vi "Loss_calc.vi"(6 "Weight Regularizers":enum32{"None", "L1", "L2"}(radio), 7 "Weights":dbl[](array[numeric]), 9 "Loss Type":enum16{"MSE", "MAE"}(ring)=enum."MAE", 10 "Target":dbl, 11 "Data":dbl) -> (3 "Loss":dbl)   [LabVIEW 2019]
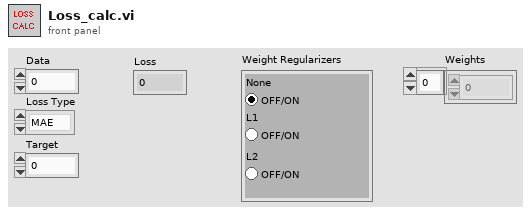
[diagram p1: front panel]
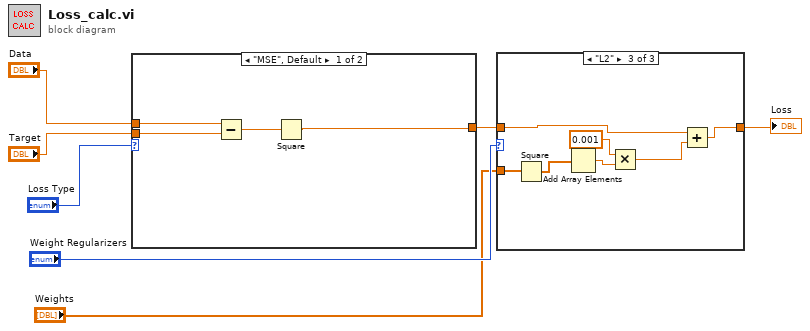
[diagram p0: block diagram]
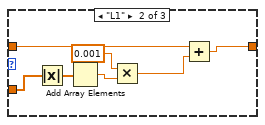
[diagram p3: hidden frame]
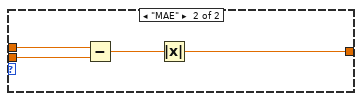
[diagram p4: hidden frame]
diagram:
  n1 = case shown="\"MSE\", Default" "Loss Type" {
    tunnel: "Data" -> [w11 w15]
    tunnel: "Target" -> [w10 w14]
    tunnel: [w8 w12] -> w3
    frame "MSE", Default {
      n2 = Subtract(x=w11, y=w10) -> (x-y=w9:dbl)
      n3 = Square(x=w9) -> (x^2=w8:dbl)
    }
    frame "MAE" {
      n4 = Subtract(x=w15, y=w14) -> (x-y=w13:dbl)
      n5 = Absolute Value(x=w13) -> (abs(x)=w12:dbl)
    }
  }
  n6 = case shown="\"L2\"" "Weight Regularizers" {
    tunnel: w3 -> [w16 w23 w27]
    tunnel: [w16 w17 w26] -> w2
    tunnel: "Weights" -> [_ w22 w25]
    frame "None", Default {
    }
    frame "L1" {
      n7 = Absolute Value(x=w22) -> (abs(x)=w18:dbl[])
      n8 = Add Array Elements(numeric array=w18) -> (sum=w19:dbl)
      n9 = Multiply(x=0.001, y=w19) -> (x*y=w20:dbl)
      n10 = Add(x=w23, y=w20) -> (x+y=w17:dbl)
    }
    frame "L2" {
      n11 = Square(x=w25) -> (x^2=w24:dbl[])
      n12 = Add Array Elements(numeric array=w24) -> (sum=w30:dbl)
      n13 = Multiply(x=0.001, y=w30) -> (x*y=w29:dbl)
      n14 = Add(x=w27, y=w29) -> (x+y=w26:dbl)
    }
  }
  "Loss" <- w2
